vi "attribute_cache_read.vi"(7 "Attribute":T1={"Identifier"="", "Descriptive name"="", "Data Type"=enum."Integer 32", "Command"="", "Access"=2, "Range Table"="", "Read Callback"="", "Write Callback"="", "Range Callback"="", "Check Callback"="", "Rngtable Callback"="", "Coerce Callback"="", "Supported Models"="", "Instrument Options"="", "Repeated Capabilities"="", "Check Status Callback"="", "Index"=0, "Flag: OPC Wait"=FALSE, "Flag: Dont check status"=FALSE, "Flag: Cache Only"=FALSE} {"Access" items=["Read Only", "Write Only", "Read/Write"]}, 8 "error in":errorcluster, 9 "Direct Attribute ID (Attribute cluster)":string, 11 "VISA resource name":refnum<visa-resource-name>) -> (0 "error out":errorcluster, 1 "Integer 32 out":i32, 2 "Double out":dbl, 3 "VISA resource name out":refnum<visa-resource-name>, 4 "String out":string, 5 "Integer 64 out":i64, 6 "Boolean out":bool, 10 "Exists in cache":bool)   [LabVIEW 2014, in "rszvl_rsidr_core.lvlib"]
uses:
  rszvl_rsidr_core.lvlib
  type_Attribute.ctl
  type_Attribute_Data_Type.ctl
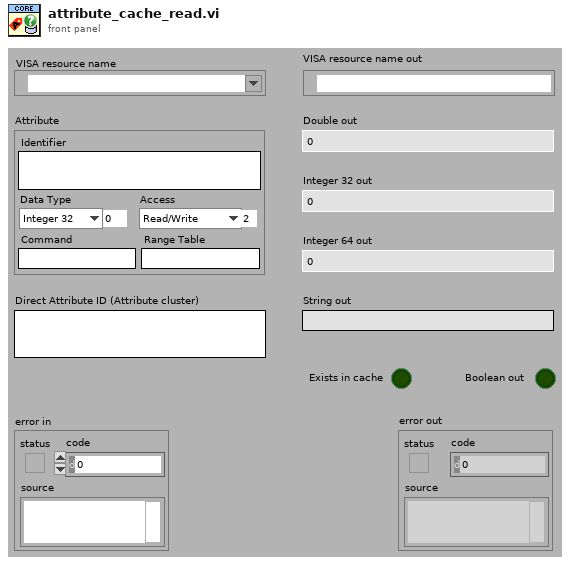
[diagram p1: front panel]
types:
  T1 = typedef "rszvl_rsidr_core.lvlib/type_Attribute.ctl" = cluster{"Identifier":string, "Descriptive name":string, "Data Type":T2, "Command":string, "Access":u16, "Range Table":string, "Read Callback":string, "Write Callback":string, "Range Callback":string, "Check Callback":string, "Rngtable Callback":string, "Coerce Callback":string, "Supported Models":string, "Instrument Options":string, "Repeated Capabilities":string, "Check Status Callback":string, "Index":i32, "Flag: OPC Wait":bool, "Flag: Dont check status":bool, "Flag: Cache Only":bool}
  T2 = typedef "rszvl_rsidr_core.lvlib/type_Attribute_Data_Type.ctl" = enum16{"Integer 32", "Double", "String", "Boolean", "None", "Integer 64"}
  T3 = enum16{"Initialize", "Get Cached Value", "Set Cached Value", "Clear"}
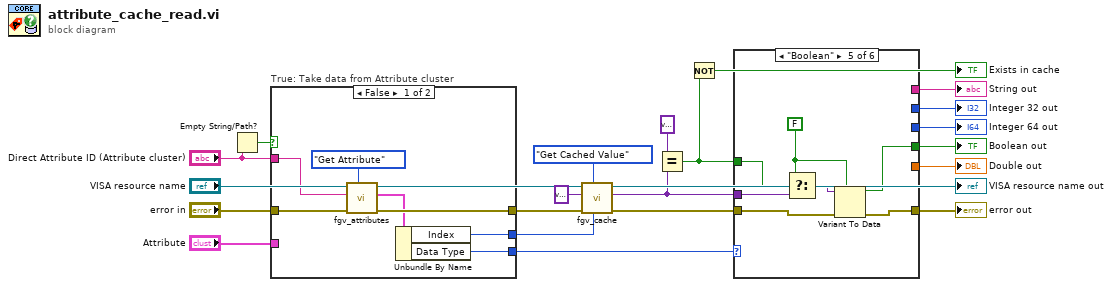
[diagram p0: block diagram]
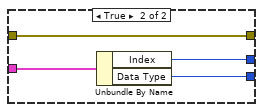
[diagram p2: hidden frame]
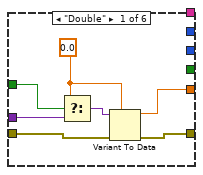
[diagram p3: hidden frame]
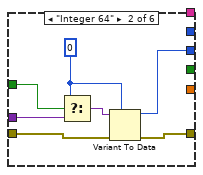
[diagram p4: hidden frame]
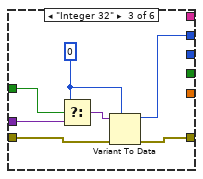
[diagram p5: hidden frame]
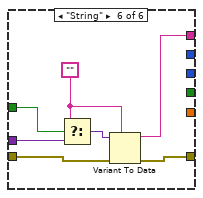
[diagram p7: hidden frame]
diagram:
  n1 = Empty String/Path?(string/path="Direct Attribute ID (Attribute cluster)") -> (empty?=w8:bool)
  n2 = case "True: Take data from Attribute cluster" shown="False" w8 {
    tunnel: "Direct Attribute ID (Attribute cluster)" -> [w26 _]
    tunnel: "error in" -> [w28 w30]
    tunnel: [w27 w30] -> w5
    tunnel: "Attribute" -> [_ w33]
    tunnel: [w25 w32] -> w2
    tunnel: [w24 w31] -> w1
    frame False {
      n3 = call "fgv_attributes.vi"("Operation"=enum16{"Initialize", "Get Attribute"}."Get Attribute", "error in"=w28, "Attribute ID in"=w26) -> ("error out"=w27:errorcluster, "Attribute out"=w23:T1)  [unwired: 6 in, 1 out]
      n4 = Unbundle By Name(w23) -> ("Index"=w25:i32, "Data Type"=w24:T2)
    }
    frame True {
      n5 = Unbundle By Name(w33) -> ("Index"=w32:i32, "Data Type"=w31:T2)
    }
  }
  n6 = call "fgv_cache.vi"("Index in"=w2, "Operation"=T3."Get Cached Value" ("Operation (1: Get Cached Value)"), "error in"=w5, "Value in"=variant, "VISA resource name"="VISA resource name") -> ("error out"=w20:errorcluster, "Cache Value out"=w15:variant, "VISA resource name out"=→"VISA resource name out":refnum<visa-resource-name>)  [unwired: 4 in]
  n7 = Equal?(x=variant ("Value"), y=w15) -> (x = y?=w14:bool)
  n8 = Not(x=w14) -> (.not. x?=→"Exists in cache":bool)
  n9 = case shown="\"Boolean\"" w1 {
    tunnel: w15 -> [w36 w43 w50 _ w58 w65]
    tunnel: w20 -> [w38 w45 w52 w55 w60 w67]
    tunnel: [w37 w44 w51 w55 w59 w66] -> w18
    tunnel: [w35 _ _ _ _ _] -> w19
    tunnel: w14 -> [w34 w42 w49 _ w57 w64]
    tunnel: [_ _ _ _ w56 _] -> w13
    tunnel: [_ _ _ _ _ w63] -> w12
    tunnel: [_ w41 _ _ _ _] -> w11
    tunnel: [_ _ w48 _ _ _] -> w10
    frame "Double" {
      w40 = 0.0 ("type")
      n10 = Select(t=w40, s=w34, f=w36) -> (s? t:f=w39:variant)
      n11 = Variant To Data(error in=w38, type=w40, Variant=w39) -> (data=w35:dbl, error out=w37:errorcluster)
    }
    frame "Integer 64" {
      w47 = i64 0 ("type")
      n12 = Select(t=w47, s=w42, f=w43) -> (s? t:f=w46:variant)
      n13 = Variant To Data(error in=w45, type=w47, Variant=w46) -> (data=w41:i64, error out=w44:errorcluster)
    }
    frame "Integer 32" {
      w54 = 0 ("type")
      n14 = Select(t=w54, s=w49, f=w50) -> (s? t:f=w53:variant)
      n15 = Variant To Data(error in=w52, type=w54, Variant=w53) -> (data=w48:i32, error out=w51:errorcluster)
    }
    frame "None" {
    }
    frame "Boolean" {
      w62 = FALSE
      n16 = Select(t=w62, s=w57, f=w58) -> (s? t:f=w61:variant)
      n17 = Variant To Data(error in=w60, type=w62, Variant=w61) -> (data=w56:bool, error out=w59:errorcluster)
    }
    frame "String" {
      w69 = "" ("type")
      n18 = Select(t=w69, s=w64, f=w65) -> (s? t:f=w68:variant)
      n19 = Variant To Data(error in=w67, type=w69, Variant=w68) -> (data=w63:string, error out=w66:errorcluster)
    }
  }
  "error out" <- w18
  "Double out" <- w19
  "Integer 64 out" <- w11
  "Integer 32 out" <- w10
  "String out" <- w12
  "Boolean out" <- w13
